vi "Read.vi"(8 "error in":errorcluster, 11 "tcp server in":refnum<class "RT FlexRIO Server TCP.lvclass">) -> (0 "error out":errorcluster, 3 "tcp server out":refnum<class "RT FlexRIO Server TCP.lvclass">)   [LabVIEW 2017, in "RT FlexRIO Server TCP.lvclass"]
uses:
  RT FlexRIO Server TCP.lvclass
  Properties/IncomingQueue_GET.vi
  Properties/Connection_GET.vi
  Properties/State_GET.vi
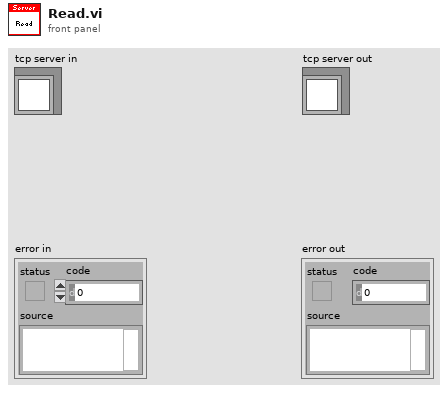
[diagram p1: front panel]
types:
  T1 = typedef "RT FlexRIO Server TCP.lvclass/State.ctl" = enum16{"started", "connected", "stopped"}
  T2 = enum16{"Standard", "Buffered", "CRLF", "Immediate"}
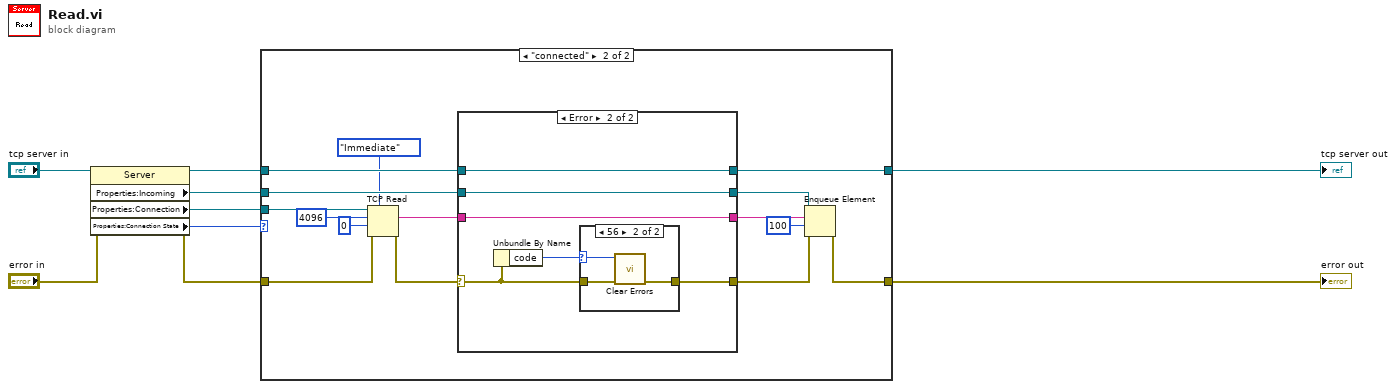
[diagram p0: block diagram]
diagram:
  n1 = property class="Server"(reference="tcp server in", error in="error in") -> (reference out=w6:refnum<class "RT FlexRIO Server TCP.lvclass">, error out=w5:errorcluster, "Properties:Incoming"=w2:refnum<queue>, "Properties:Connection"=w3:refnum<k5>, "Properties:Connection State"=w1:T1)
  n2 = case shown="\"connected\"" w1 {
    tunnel: w6 -> [w11 w24]
    tunnel: [w10 w12] -> w8
    tunnel: [w11 w25] -> w7
    tunnel: w5 -> [w10 w19]
    tunnel: w3 -> [_ w20]
    tunnel: w2 -> [_ w26]
    frame "started", Default {
    }
    frame "connected" {
      n3 = TCP Read(connection ID=w20, bytes to read=4096, error in (no error)=w19, 7:T2."Immediate" ("mode (standard)"), 9:0 ("timeout ms (25000)")) -> (data out=w17:string, error out=w18:errorcluster)  [unwired: 1 out]
      n4 = case shown="Error" w18 {
        selector: w18 -> [w27 w35]
        tunnel: [w27 w33] -> w13
        tunnel: w26 -> [w29 w32]
        tunnel: [w30 w34] -> w25
        tunnel: w24 -> [w30 w34]
        tunnel: w17 -> [w28 w31]
        tunnel: [w29 w32] -> w15
        tunnel: [w28 w31] -> w14
        frame No Error {
        }
        frame Error {
          n5 = Unbundle By Name(w35) -> ("code"=w36:i32)
          n6 = case shown="56" w36 {
            selector: w36 -> [_ w38]
            tunnel: [w37 w39] -> w33
            tunnel: w35 -> [w37 w40]
            frame 0, Default {
            }
            frame 56 {
              n7 = call <vilib>:"Clear Errors.vi"("error in (no error)"=w40, "specific error code to clear (0: all)"=w38) -> ("error out"=w39:errorcluster)  [unwired: 4 in, 1 out]
            }
          }
        }
      }
      n8 = Enqueue Element(queue=w15, element=w14, timeout in ms (-1)=100, error in (no error)=w13) -> (error out=w12:errorcluster)  [unwired: 2 out]
    }
  }
  "error out" <- w8
  "tcp server out" <- w7
